vi "Write Value.vi"(8 "error in (no error)":errorcluster, 9 "Value":u16 format="%04x", 10 "Index":i32, 11 "Virtual Memory Unit in":refnum<class "Virtual Memory Unit.lvclass">) -> (0 "error out":errorcluster, 3 "Virtual Memory Unit out":refnum<class "Virtual Memory Unit.lvclass">)   [LabVIEW 2020, in "BCI-1553 API.lvlib" / "Virtual Memory.lvlib" / "Virtual Memory Unit.lvclass"]
doc: "Write a single value into memory."
uses:
  Virtual Memory Unit.lvclass
  Virtual Memory Unit.lvclass/Virtual Memory Unit.ctl
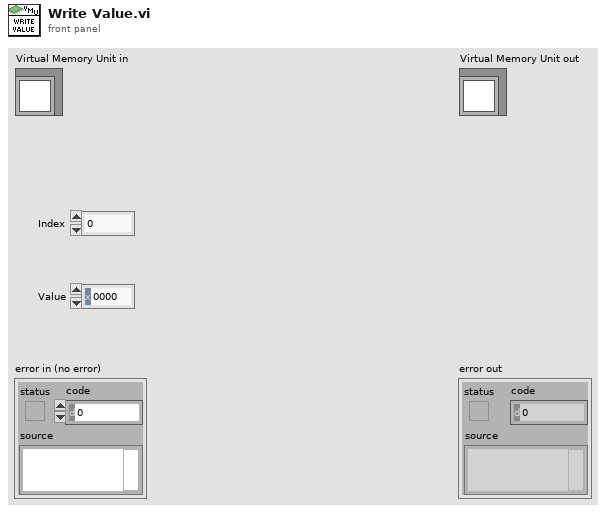
[diagram p1: front panel]
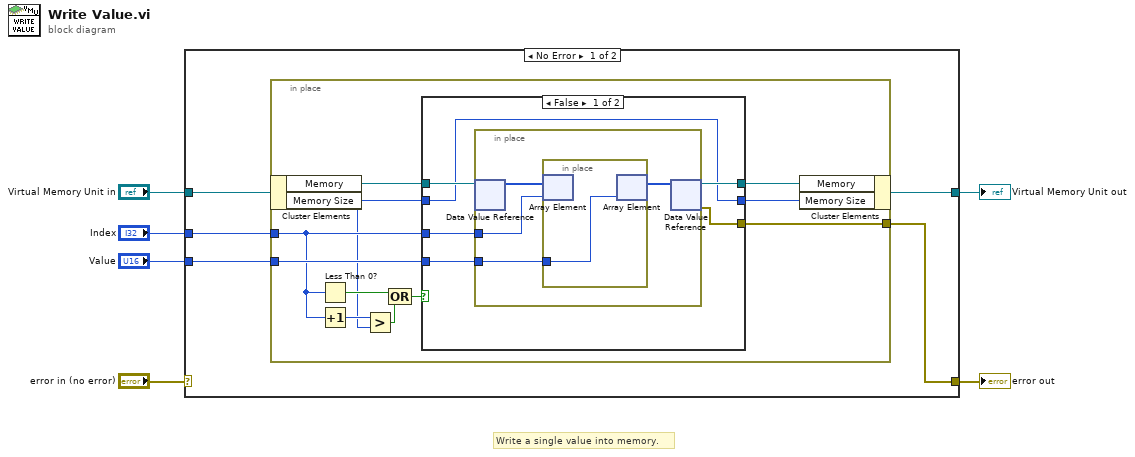
[diagram p0: block diagram]
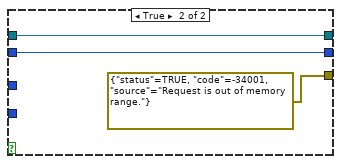
[diagram p2: hidden frame]
diagram:
  # "Write a single value into memory."
  n1 = case shown="No Error" "error in (no error)" {
    selector: "error in (no error)" -> [_ w38]
    tunnel: [w7 w38] -> w5
    tunnel: [w10 w37] -> w3
    tunnel: "Virtual Memory Unit in" -> [w11 w37]
    tunnel: "Index" -> [w9 _]
    tunnel: "Value" -> [w8 _]
    frame No Error {
      n2 = in-place {
        in-place-border: w9 -> [w14]
        in-place-border: w8 -> [w21]
        in-place-border: [w19] -> w7
        n3 = in-place-cluster #1(w11) -> ("Memory"=w22:refnum<data-value>, "Memory Size"=w12:i32)
        n4 = Less Than 0?(x=w14) -> (x < 0?=w17:bool)
        n5 = Increment(x=w14) -> (x+1=w13:i32)
        n6 = Greater?(x=w13, y=w12) -> (0:w16:bool)
        n7 = Compound Arithmetic op=OR(w17, w16) -> (w15:bool)
        n8 = case shown="False" w15 {
          tunnel: w22 -> [w28 w36]
          tunnel: w14 -> [w27 _]
          tunnel: w21 -> [w26 _]
          tunnel: [w25 w36] -> w20
          tunnel: [w24 errorcluster {"status"=TRUE, "code"=-34001, "source"="Request is out of memory range."} ("error IO")] -> w19
          tunnel: [w23 w35] -> w18
          tunnel: w12 -> [w23 w35]
          frame False {
            n9 = in-place {
              in-place-border: w27 -> [w31]
              in-place-border: w26 -> [w30]
              n10 = in-place-dvr #2(w28) -> (w32:u16[])  [unwired: 1 out]
              n11 = in-place {
                in-place-border: w30 -> [w33]
                n12 = in-place-array #3(w32, w31) -> ()  [unwired: 1 out]
                n13 = in-place-array #3(w33) -> (w29:u16[])  [unwired: 1 out]
              }
              n14 = in-place-dvr #2(w29) -> (w25:refnum<data-value>, w24:errorcluster)
            }
          }
          frame True {
          }
        }
        n15 = in-place-cluster #1("Memory"=w20, "Memory Size"=w18) -> (w10:refnum<class "Virtual Memory Unit.lvclass">)
      }
    }
    frame Error {
    }
  }
  "error out" <- w5
  "Virtual Memory Unit out" <- w3
